vi "Populate Filenames.vi"(8 "error in":errorcluster, 11 "UI Actor in":refnum<class "UI Actor.lvclass">) -> (0 "error out":errorcluster)   [LabVIEW 2019, in "UI Actor.lvlib" / "UI Actor.lvclass"]
uses:
  UI Actor.lvclass
  UI Actor.lvclass/UI Actor.ctl
  Electronic Datasheet/Electronic Datasheet.lvclass
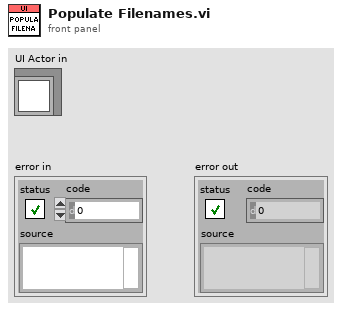
[diagram p1: front panel]
types:
  T1 = map{path, refnum<class "Electronic Datasheet.lvclass">}
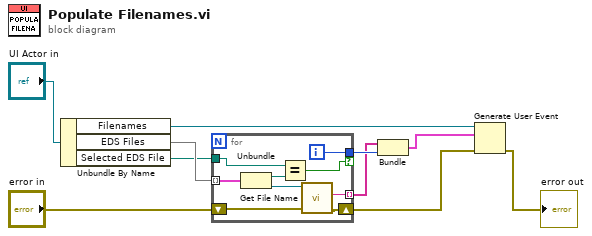
[diagram p0: block diagram]
diagram:
  n1 = Unbundle By Name("UI Actor in") -> ("Filenames"=w8:refnum<user-event>, "EDS Files"=w5:T1, "Selected EDS File"=w4:path)
  n2 = for {
    tunnel: w5 -> [w19] mode=indexing
    tunnel: [w17] -> w2 mode=indexing
    shift-right: [w15] -> w10
    shift-left: "error in" -> [w16]
    tunnel: w4 -> [w14]
    tunnel: [w12] -> w3 if=w11
    i -> [w12]
    n3 = Unbundle(w19) -> ("File Path"=w13:path, "EDS"=w18:refnum<class "Electronic Datasheet.lvclass">)
    n4 = Equal?(x=w14, y=w13) -> (x = y?=w11:bool)
    n5 = call "Get File Name.vi"("error in"=w16, "reference in"=w18) -> ("error out"=w15:errorcluster, "File Name"=w17:string)  [unwired: 7 in, 1 out]
  }
  n6 = Bundle(w2, w3) -> (w1:cluster{string[], i32})  [unwired: 1 in]
  n7 = Generate User Event(user event=w8, event data cluster=w1, error in=w10) -> (error out=→"error out":errorcluster)  [unwired: 1 in, 1 out]
